vi "CB Get Motor Values.vi"(6 "k":dbl=1.0, 9 "num motors":i32=1, 11 "Motor ID":T1) -> (1 "Kt":dbl, 2 "Kv":dbl, 3 "R":dbl, 4 "motor properities (single)":T2)   [LabVIEW 2020]
uses:
  CB Motor ID.ctl
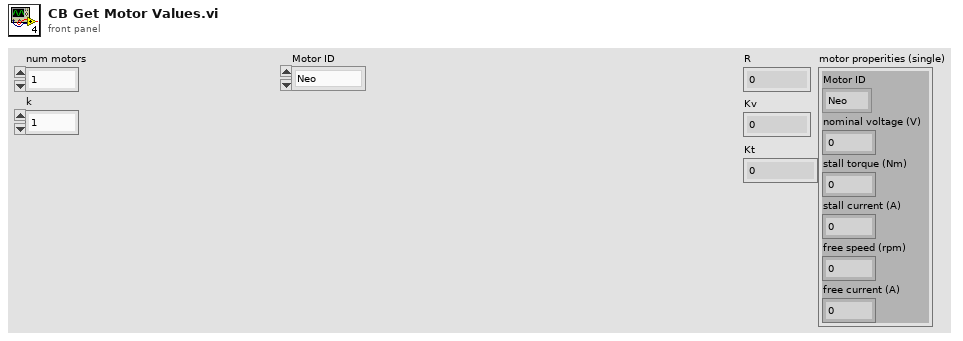
[diagram p1: front panel]
types:
  T1 = typedef "CB Motor ID.ctl" = enum16{"Neo", "Neo 550", "Falcon 500", "775pro"}
  T2 = cluster{"Motor ID":T1, "nominal voltage (V)":dbl, "stall torque (Nm)":dbl, "stall current (A)":dbl, "free speed (rpm)":dbl, "free current (A)":dbl}
  T3 = cluster{"Motor ID":T1, "nominal voltage (V)":dbl, "stall torque (Nm)":dbl, "stall current (A)":dbl, "free speed (rpm)":dbl, "free current (A)":dbl}[]
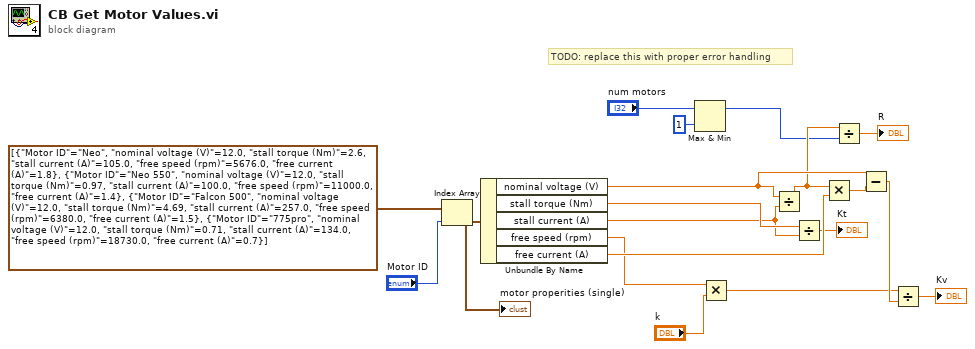
[diagram p0: block diagram]
diagram:
  # "TODO: replace this with proper error handling"
  n1 = Index Array(array=T3 [{"Motor ID"=enum."Neo", "nominal voltage (V)"=12.0, "stall torque (Nm)"=2.6, "stall current (A)"=105.0, "free speed (rpm)"=5676.0, "free current (A)"=1.8}, {"Motor ID"=enum."Neo 550", "nominal voltage (V)"=12.0, "stall torque (Nm)"=0.97, "stall current (A)"=100.0, "free speed (rpm)"=11000.0, "free current (A)"=1.4}, {"Motor ID"=enum."Falcon 500", "nominal voltage (V)"=12.0, "stall torque (Nm)"=4.69, "stall current (A)"=257.0, "free speed (rpm)"=6380.0, "free current (A)"=1.5}, {"Motor ID"=enum."775pro", "nominal voltage (V)"=12.0, "stall torque (Nm)"=0.71, "stall current (A)"=134.0, "free speed (rpm)"=18730.0, "free current (A)"=0.7}] ("appended array"), index="Motor ID") -> (element=w17:T2)
  "motor properities (single)" <- w17
  n2 = Unbundle By Name(w17) -> ("nominal voltage (V)"=w12:dbl, "stall torque (Nm)"=w16:dbl, "stall current (A)"=w15:dbl, "free speed (rpm)"=w3:dbl, "free current (A)"=w14:dbl)
  n3 = Max & Min(x="num motors", y=1) -> (max(x,y)=w5:i32)  [unwired: 1 out]
  n4 = Multiply(x=w3, y="k") -> (x*y=w1:dbl)
  n5 = Divide(x=w12, y=w15) -> (x/y=w6:dbl)
  n6 = Divide(x=w16, y=w15) -> (x/y=→"Kt":dbl)
  n7 = Multiply(x=w6, y=w14) -> (x*y=w13:dbl)
  n8 = Divide(x=w6, y=w5) -> (x/y=→"R":dbl)
  n9 = Subtract(x=w12, y=w13) -> (x-y=w11:dbl)
  n10 = Divide(x=w1, y=w11) -> (x/y=→"Kv":dbl)
